vi "Get Server Port Number.vi"(8 "error in (no error)":errorcluster, 11 "Target LV Version #":T1) -> (0 "error out":errorcluster, 2 "Version Number":string, 3 "Server Port":u16)   [LabVIEW 2016]
uses:
  Sub Controls/LV Versions Enum.ctl
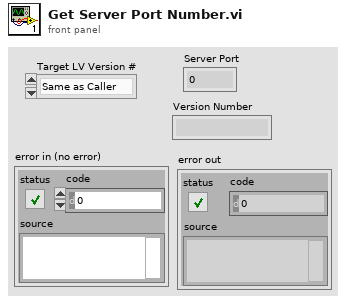
[diagram p1: front panel]
types:
  T1 = typedef "LV Versions Enum.ctl" = enum16{"Same as Caller", "8.0", "8.20", "8.5", "8.6", "9.0", "10.0", "11.0", "12.0", "13.0", "14.0", "15.0", "16.0", "17.0", "18.0", "19.0", "20.0"}
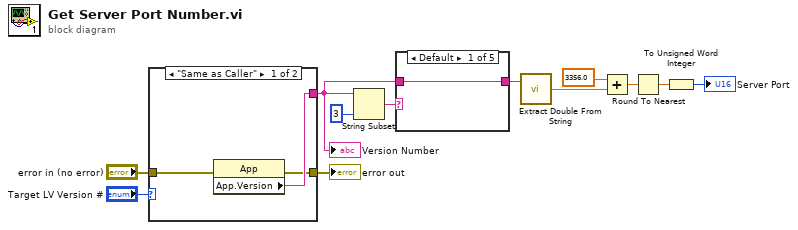
[diagram p0: block diagram]
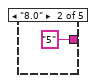
[diagram p2: hidden frame]
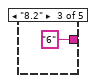
[diagram p3: hidden frame]
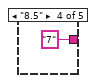
[diagram p4: hidden frame]
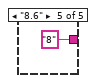
[diagram p5: hidden frame]
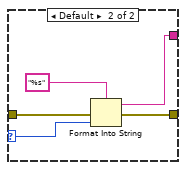
[diagram p6: hidden frame]
diagram:
  n1 = case shown="\"Same as Caller\"" "Target LV Version #" {
    selector: "Target LV Version #" -> [_ w19]
    tunnel: [w15 w18] -> w1
    tunnel: "error in (no error)" -> [w14 w16]
    tunnel: [w13 w17] -> w6
    frame "Same as Caller" {
      n2 = property class="App"(error in=w14) -> (error out=w13:errorcluster, "App.Version"=w15:string)  [unwired: 1 in, 1 out]
    }
    frame Default {
      n3 = Format Into String(format string="%s", error in=w16, w19) -> (resulting string=w18:string, error out=w17:errorcluster)  [unwired: 1 in]
    }
  }
  "Version Number" <- w1
  "error out" <- w6
  n4 = String Subset(string=w1, length (rest)=3 ("length (rest)")) -> (substring=w3:string)  [unwired: 1 in]
  n5 = case shown="Default" w3 {
    tunnel: [w21 "5" ("regular expression") "6" ("regular expression") "7" ("regular expression") "8" ("regular expression")] -> w2
    tunnel: w1 -> [w21 _ _ _ _]
    frame Default {
    }
    frame "8.0" {
    }
    frame "8.2" {
    }
    frame "8.5" {
    }
    frame "8.6" {
    }
  }
  n6 = call "Extract Double From String.vi"("string"=w2) -> ("floating pt. number"=w12:dbl)  [unwired: 1 in, 2 out]
  n7 = Add(x=3356.0, y=w12) -> (x+y=w10:dbl)
  n8 = Round To Nearest(number=w10) -> (nearest integer value=w9:dbl)
  n9 = To Unsigned Word Integer(number=w9) -> (unsigned 16bit integer=→"Server Port":u16)
